vi "_session_get_additionalFlag_value.vi"(3 "AdditionalFlags value in":i32 format="%011b", 5 "AdditionalFlag bit":T1) -> (1 "AdditionalFlag bit value out":bool)   [LabVIEW 2020, in "Rohde&Schwarz RTx Oscilloscopes.lvlib" / "rsidr_core.lvlib"]
uses:
  rsidr_core.lvlib
  type_AdditionalFlag_Bits.ctl
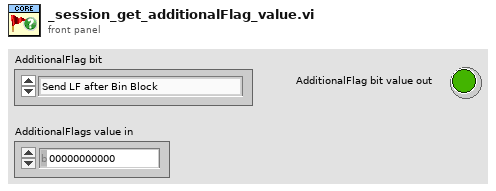
[diagram p1: front panel]
types:
  T1 = typedef "Rohde&Schwarz RTx Oscilloscopes.lvlib/rsidr_core.lvlib/type_AdditionalFlag_Bits.ctl" = enum16{"Send LF after Bin Block", "Junk read with io_clear_buffers.vi", "io_clear_buffers: viClear()", "io_clear_buffers: viFlush()", "<NotUsed1>", "Allow Dbl & Int Bin/Ascii read", "*OPC? in check_instrument_error.vi", "<NotUsed2>", "Smart Enum Matching", "Less Strict RepCaps check", "AssureResponseEndWithLF"}
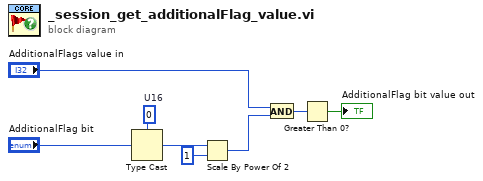
[diagram p0: block diagram]
diagram:
  w7 = u16 0  # U16
  n1 = Type Cast(type=w7, x="AdditionalFlag bit") -> (*(type *) &x=w6:u16)
  n2 = Scale By Power Of 2(n=w6, x=1) -> (x*2^n=w3:i32)
  n3 = And(x="AdditionalFlags value in", y=w3) -> (x .and. y?=w2:i32)
  n4 = Greater Than 0?(x=w2) -> (x > 0?=→"AdditionalFlag bit value out":bool)
